vi "sub_path_position.vi"   [LabVIEW 2019]
uses:
  Ctrl/waypoint_buf.ctl
types:
  T1 = typedef "waypoint_buf.ctl" = enum16{"clear", "write", "read"}
  T2 = cluster{"lookahead pt n":dbl, "lookahead distance":dbl}
  T3 = cluster{"incircle wpt":cluster{dbl, dbl}[], "agv circle":cluster{dbl, dbl}[], "offset":cluster{dbl, dbl}[], "lookahead":cluster{"x":dbl, "y":dbl}[], "looktail":cluster{"x":dbl, "y":dbl}[]}
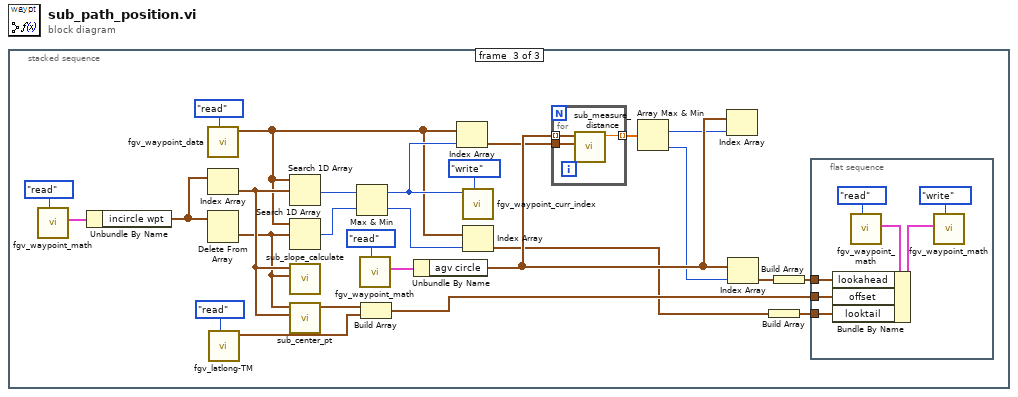
[diagram p0: block diagram]
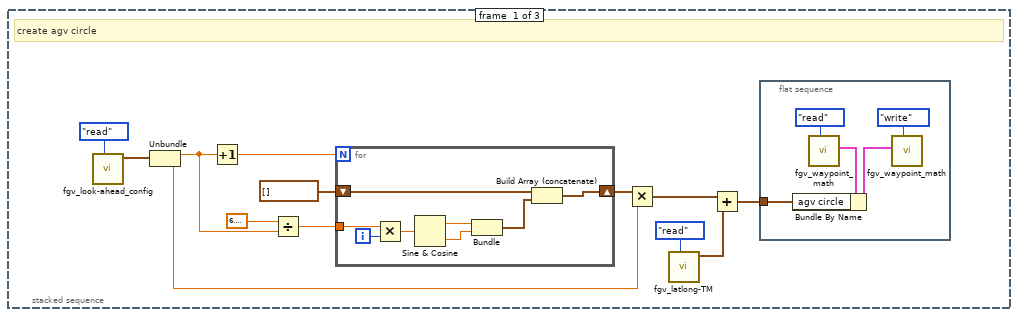
[diagram p2: hidden frame]
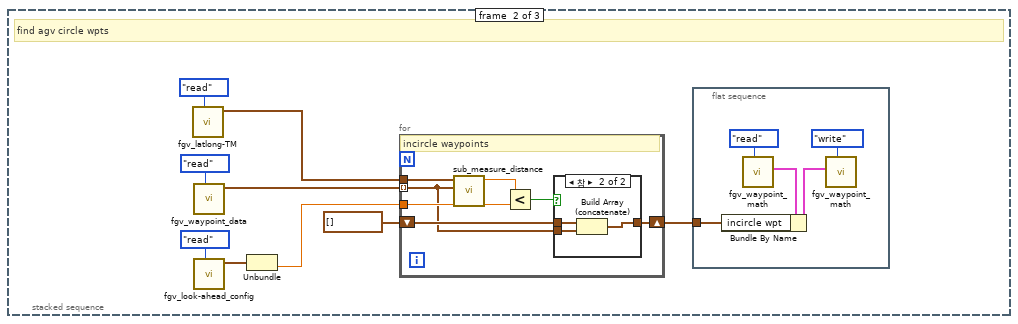
[diagram p3: hidden frame]
diagram:
  n1 = stacked-sequence {
    frame #0 {
      # "create agv circle"
      n2 = call "fgv_look-ahead_config.vi"("cmd"=enum16{"read", "write"}."read") -> ("lookahed cfg out"=w11:T2)  [unwired: 10 in]
      n3 = Unbundle(w11) -> ("lookahead pt n"=w10:dbl, "lookahead distance"=w9:dbl)
      n4 = Increment(x=w10) -> (x+1=w12:dbl)
      n5 = Divide(x=6.283185307179586, y=w10) -> (x/y=w13:dbl)
      n6 = for {
        N: w12 -> [_]
        tunnel: w13 -> [w22]
        shift-right: [w24] -> w6
        shift-left: cluster{dbl, dbl}[] [] -> [w23]
        i -> [w21]
        n7 = Multiply(x=w22, y=w21) -> (x*y=w20:dbl)
        n8 = Sine & Cosine(0:w20) -> (1:w25:dbl, 2:w26:dbl)
        n9 = Bundle(w25, w26) -> (w19:cluster{dbl, dbl})  [unwired: 1 in]
        n10 = Build Array (concatenate)(w23, w19) -> (w24:cluster{dbl, dbl}[])
      }
      n11 = Multiply(x=w6, y=w9) -> (x*y=w8:cluster{dbl, dbl}[])
      n12 = call "fgv_latlong-TM.vi"("cmd"=enum16{"write", "read"}."read") -> ("latlong out"=w7:cluster{"lat":dbl, "long":dbl})  [unwired: 9 in, 1 out]
      n13 = Add(x=w8, y=w7) -> (x+y=w1:cluster{dbl, dbl}[])
      n14 = flat-sequence {
        tunnel: w1 -> [w14]
        frame #0 {
          n15 = call "fgv_waypoint_math.vi"("cmd"=waypoint_buf."read") -> ("wpt data"=w17:T3)  [unwired: 9 in, 1 out]
          n16 = Bundle By Name(cluster=w17, "agv circle"=w14) -> (w18:T3)
          n17 = call "fgv_waypoint_math.vi"("cmd"=waypoint_buf."write", "wpt data"=w18) -> ()  [unwired: 8 in, 2 out]
        }
      }
    }
    frame #1 {
      # "find agv circle wpts"
      n18 = call "fgv_latlong-TM.vi"("cmd"=enum16{"write", "read"}."read") -> ("latlong out"=w29:cluster{"lat":dbl, "long":dbl})  [unwired: 9 in, 1 out]
      n19 = call "fgv_waypoint_data.vi"("cmd"=waypoint_buf."read") -> ("waypoint out"=w33:cluster{"x":dbl, "y":dbl}[])  [unwired: 8 in, 2 out]
      n20 = call "fgv_look-ahead_config.vi"("cmd"=enum16{"read", "write"}."read") -> ("lookahed cfg out"=w31:T2)  [unwired: 10 in]
      n21 = Unbundle(w31) -> ("lookahead distance"=w32:dbl)  [unwired: 1 out]
      n22 = for {
        tunnel: w33 -> [w42] mode=indexing
        tunnel: w29 -> [w47]
        shift-right: [w41] -> w34
        shift-left: cluster{"x":dbl, "y":dbl}[] [] -> [w44]
        tunnel: w32 -> [w45]
        # "incircle waypoints"
        n23 = call "sub_measure_distance.vi"("pt 2"=w42, "pt 1"=w47) -> ("distance"=w46:dbl)  [unwired: 9 in]
        n24 = Less?(x=w46, y=w45) -> (x < y?=w43:bool)
        n25 = case shown="참" w43 {
          tunnel: w44 -> [w48 w51]
          tunnel: w42 -> [_ w50]
          tunnel: [w48 w49] -> w41
          frame False {
          }
          frame True {
            n26 = Build Array (concatenate)(w51, w50) -> (w49:cluster{"x":dbl, "y":dbl}[])
          }
        }
      }
      n27 = flat-sequence {
        tunnel: w34 -> [w40]
        frame #0 {
          n28 = call "fgv_waypoint_math.vi"("cmd"=waypoint_buf."read") -> ("wpt data"=w38:T3)  [unwired: 9 in, 1 out]
          n29 = Bundle By Name(cluster=w38, "incircle wpt"=w40) -> (w39:T3)
          n30 = call "fgv_waypoint_math.vi"("cmd"=waypoint_buf."write", "wpt data"=w39) -> ()  [unwired: 8 in, 2 out]
        }
      }
    }
    frame #2 {
      n31 = call "fgv_waypoint_math.vi"("cmd"=waypoint_buf."read") -> ("wpt data"=w55:T3)  [unwired: 9 in, 1 out]
      n32 = Unbundle By Name(w55) -> ("incircle wpt"=w54:cluster{dbl, dbl}[])
      n33 = call "fgv_waypoint_data.vi"("cmd"=waypoint_buf."read") -> ("waypoint out"=w64:cluster{"x":dbl, "y":dbl}[])  [unwired: 8 in, 2 out]
      n34 = Index Array(array=w54) -> (element=w76:cluster{dbl, dbl})  [unwired: 1 in]
      n35 = Delete From Array(array=w54) -> (deleted portion=w75:cluster{dbl, dbl})  [unwired: 2 in, 1 out]
      n36 = call "fgv_latlong-TM.vi"("cmd"=enum16{"write", "read"}."read") -> ("latlong out"=w65:cluster{"lat":dbl, "long":dbl})  [unwired: 9 in, 1 out]
      n37 = Search 1D Array(1D array=w64, element=w76) -> (index of element=w71:i32)  [unwired: 1 in]
      n38 = Search 1D Array(1D array=w64, element=w75) -> (index of element=w72:i32)  [unwired: 1 in]
      n39 = call "sub_slope_calculate.vi"("point n+1"=w75, "point n"=w76) -> ()  [unwired: 7 in, 3 out]
      n40 = call "sub_center_pt.vi"("point-2"=w76, "point-1"=w75) -> ("center"=w66:cluster{"x":dbl, "y":dbl})  [unwired: 9 in]
      n41 = Max & Min(x=w71, y=w72) -> (max(x,y)=w74:i32, min(x,y)=w73:i32)
      n42 = call "fgv_waypoint_math.vi"("cmd"=waypoint_buf."read") -> ("wpt data"=w77:T3)  [unwired: 9 in, 1 out]
      n43 = Build Array(w66, w65) -> (w57:cluster{"lat":dbl, "long":dbl}[])
      n44 = Unbundle By Name(w77) -> ("agv circle"=w78:cluster{dbl, dbl}[])
      n45 = Index Array(array=w64, index=w74) -> (element=w67:cluster{"x":dbl, "y":dbl})
      n46 = call "fgv_waypoint_curr_index.vi"("cmd"=enum16{"write", "read"}."write", "index in"=w74) -> ()  [unwired: 9 in, 1 out]
      n47 = Index Array(array=w64, index=w73) -> (element=w53:cluster{"x":dbl, "y":dbl})
      n48 = for {
        tunnel: w78 -> [w88] mode=indexing
        tunnel: w67 -> [w87]
        tunnel: [w86] -> w68 mode=indexing
        n49 = call "sub_measure_distance.vi"("pt 2"=w87, "pt 1"=w88) -> ("distance"=w86:dbl)  [unwired: 9 in]
      }
      n50 = Array Max & Min(array=w68) -> (max index (indices)=w70:i32, min index (indices)=w69:i32)  [unwired: 2 out]
      n51 = Index Array(array=w78, index=w70) -> ()  [unwired: 1 out]
      n52 = Index Array(array=w78, index=w69) -> (element=w58:cluster{dbl, dbl})
      n53 = Build Array(w53) -> (w52:cluster{"x":dbl, "y":dbl}[])
      n54 = Build Array(w58) -> (w56:cluster{dbl, dbl}[])
      n55 = flat-sequence {
        tunnel: w56 -> [w81]
        tunnel: w57 -> [w80]
        tunnel: w52 -> [w79]
        frame #0 {
          n56 = call "fgv_waypoint_math.vi"("cmd"=waypoint_buf."read") -> ("wpt data"=w84:T3)  [unwired: 9 in, 1 out]
          n57 = Bundle By Name(cluster=w84, "lookahead"=w81, "offset"=w80, "looktail"=w79) -> (w85:T3)
          n58 = call "fgv_waypoint_math.vi"("cmd"=waypoint_buf."write", "wpt data"=w85) -> ()  [unwired: 8 in, 2 out]
        }
      }
    }
  }
